vi "ButtonDecrementToteCount.vi"(11 "Buttons":bool[](array[boolean])) -> ()   [LabVIEW 2014]
uses:
  ToteCount.vi
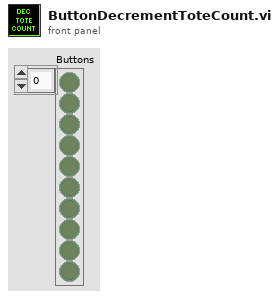
[diagram p1: front panel]
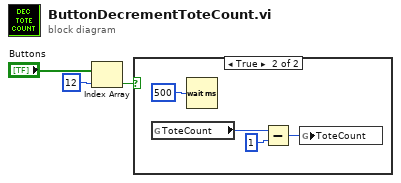
[diagram p0: block diagram]
diagram:
  n1 = Index Array(array="Buttons", index=12) -> (element=w1:bool)
  n2 = case shown="True" w1 {
    frame False {
    }
    frame True {
      n3 = global read "ToteCount.vi" "ToteCount"() -> (w5:i32)
      n4 = Wait (ms)(milliseconds to wait=u32 500) -> ()  [unwired: 1 out]
      n5 = Subtract(x=w5, y=1) -> (x-y=w6:i32)
      n6 = global write "ToteCount.vi" "ToteCount"(w6) -> ()
    }
  }
